vi "generateSignedBlobs.vi"(6 "timeout (10000)":i32=10000, 8 "error in (no error)":errorcluster, 11 "Parameters":T2={"params"={"apiKey"="", "n"=0, "size"=0, "format"="base64"}, "id"=0.0}) -> (0 "error out":errorcluster, 3 "Response":T1={"result"={"random"={"method"="", "hashedApiKey"="", "n"=0, "size"=0, "format"="base64", "data"=[], "completionTime"="", "serialNumber"=0}, "signature"="", "bitsUsed"=0, "bitsLeft"=0, "requestsLeft"=0, "advisoryDelay"=0}, "id"=0.0}, 4 "error data":string[](array[string]))   [LabVIEW 2014, in "Random JSON API.lvlib"]
uses:
  Random JSON API.lvlib
  Type Defs/generateBlobsRequest.ctl
  Type Defs/generateSignedBlobsResponse.ctl
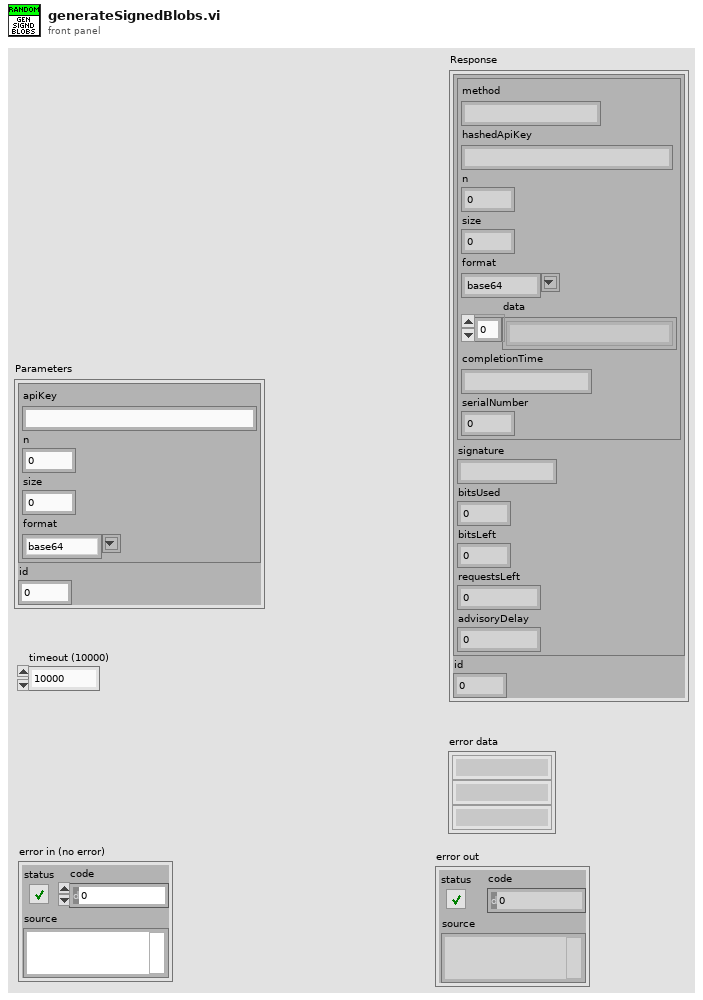
[diagram p1: front panel]
types:
  T1 = typedef "Random JSON API.lvlib/generateSignedBlobsResponse.ctl" = cluster{"result":cluster{"random":cluster{"method":string, "hashedApiKey":string, "n":i32, "size":i32, "format":string, "data":string[], "completionTime":string, "serialNumber":i32}, "signature":string, "bitsUsed":i32, "bitsLeft":i32, "requestsLeft":i32, "advisoryDelay":i32}, "id":dbl}
  T2 = typedef "Random JSON API.lvlib/generateBlobsRequest.ctl" = cluster{"params":cluster{"apiKey":string, "n":i32, "size":i32, "format":string}, "id":dbl}
  T3 = cluster{"apiKey":string, "n":i32, "size":i32, "format":string}
  T4 = cluster{"jsonrpc":string, "method":string, "params":cluster{"apiKey":string, "n":i32, "size":i32, "format":string}, "id":dbl}
  T5 = cluster{"result cluster":cluster{"completionTime":string, "bitsUsed":i32, "bitsLeft":i32, "requestsLeft":i32, "advisoryDelay":i32}, "method":string, "hashedApiKey":string, "n":i32, "serialNumber":i32, "signature":string}
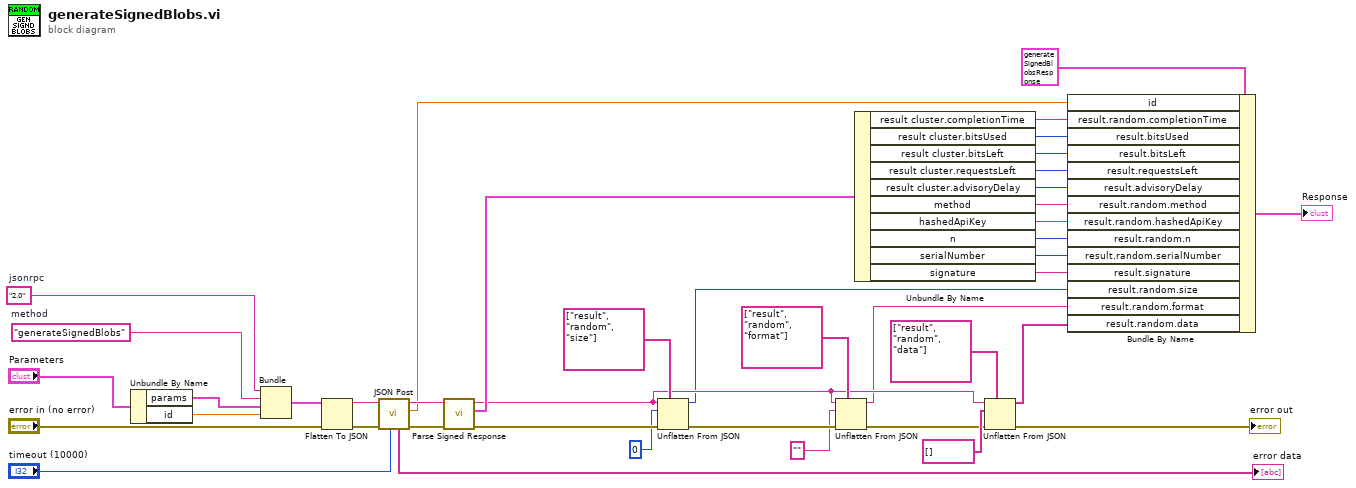
[diagram p0: block diagram]
diagram:
  w27 = "2.0"  # jsonrpc
  w32 = "generateSignedBlobs"  # method
  n1 = Unbundle By Name("Parameters") -> ("params"=w30:T3, "id"=w29:dbl)
  n2 = Bundle("jsonrpc"=w27, "method"=w32, "params"=w30, "id"=w29) -> (w28:T4)  [unwired: 1 in]
  n3 = Flatten To JSON(anything=w28, error in (no error)="error in (no error)") -> (JSON string=w33:string, 11:w34:errorcluster)  [unwired: 1 in]
  n4 = call "JSON Post.vi"("timeout (10000)"="timeout (10000)", "error in (no error)"=w34, "Request JSON String"=w33) -> ("error out"=w41:errorcluster, "id"=w25:dbl, "Response JSON String"=w26:string, "error data"=→"error data":string[])  [unwired: 5 in]
  n5 = call "Parse Signed Response.vi"("error in (no error)"=w41, "body in"=w26) -> ("error out"=w8:errorcluster, "signed result cluster"=w24:T5, "body out"=w4:string)  [unwired: 7 in]
  n6 = Unflatten From JSON(path=string[] ["result", "random", "size"], JSON string=w4, type and defaults=0, error in (no error)=w8) -> (value=w2:i32, error out=w7:errorcluster)  [unwired: 3 in]
  n7 = Unflatten From JSON(path=string[] ["result", "random", "format"], JSON string=w4, type and defaults="", error in (no error)=w7) -> (value=w3:string, error out=w6:errorcluster)  [unwired: 3 in]
  n8 = Unbundle By Name(w24) -> ("result cluster.completionTime"=w40:string, "result cluster.bitsUsed"=w39:i32, "result cluster.bitsLeft"=w38:i32, "result cluster.requestsLeft"=w37:i32, "result cluster.advisoryDelay"=w36:i32, "method"=w16:string, "hashedApiKey"=w15:string, "n"=w14:i32, "serialNumber"=w13:i32, "signature"=w12:string)
  n9 = Unflatten From JSON(path=string[] ["result", "random", "data"], JSON string=w4, type and defaults=string[] [], error in (no error)=w6) -> (value=w11:string[], error out=→"error out":errorcluster)  [unwired: 3 in]
  n10 = Bundle By Name(cluster=T1 {"result"={"random"={"method"="", "hashedApiKey"="", "n"=0, "size"=0, "format"="base64", "data"=[], "completionTime"="", "serialNumber"=0}, "signature"="", "bitsUsed"=0, "bitsLeft"=0, "requestsLeft"=0, "advisoryDelay"=0}, "id"=0.0} ("Response"), "id"=w25, "result.random.completionTime"=w40, "result.bitsUsed"=w39, "result.bitsLeft"=w38, "result.requestsLeft"=w37, "result.advisoryDelay"=w36, "result.random.method"=w16, "result.random.hashedApiKey"=w15, "result.random.n"=w14, "result.random.serialNumber"=w13, "result.signature"=w12, "result.random.size"=w2, "result.random.format"=w3, "result.random.data"=w11) -> (→"Response":T1)
